vi "Load Views.vi"(8 "error in (no error)":errorcluster, 9 "Views":refnum<class "Actor.lvclass">[](array[class]), 10 "Names":string[](array[string]), 11 "MVVM Abstruct Controller in":refnum<class "MVVM Abstruct Controller.lvclass">) -> (0 "error out":errorcluster, 3 "MVVM Abstruct Controller out":refnum<class "MVVM Abstruct Controller.lvclass">)   [LabVIEW 2020, in "MVVM Abstruct Controller.lvlib" / "MVVM Abstruct Controller.lvclass"]
uses:
  MVVM Abstruct Controller.lvclass
  C:/Program Files (x86)/National Instruments/LabVIEW 2020/vi.lib/ActorFramework/Actor/Actor.lvclass
  <vilib>/ActorFramework/Actor/Actor.lvclass
  MVVM Abstruct Controller.lvclass/MVVM Abstruct Controller.ctl
  C:/Users/yu/Desktop/Pro1/06 Source/Code/Common/ActorMap/ActorMap.lvclass
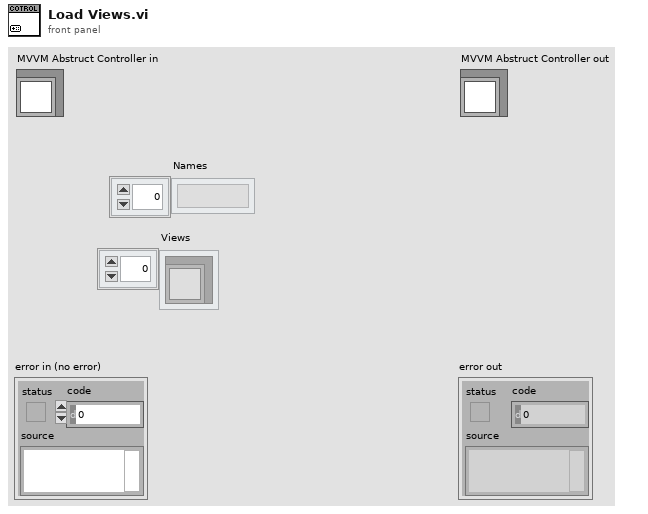
[diagram p1: front panel]
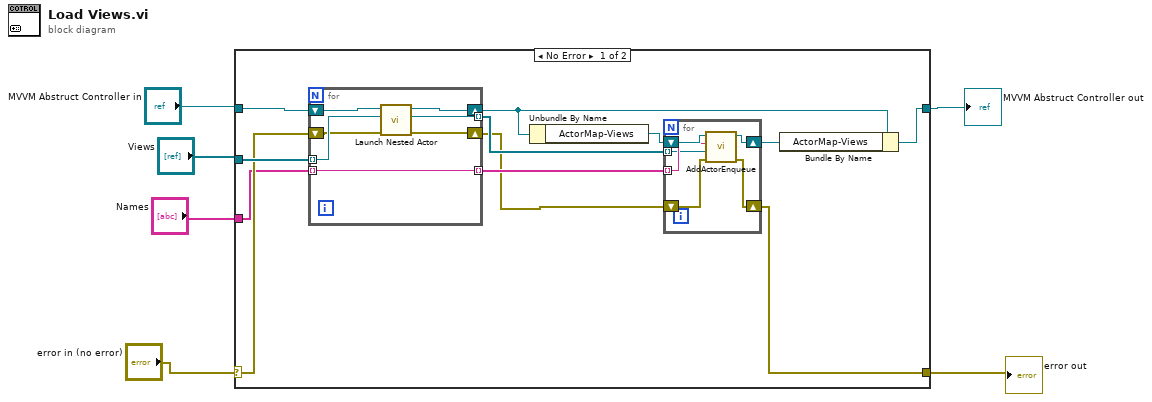
[diagram p0: block diagram]
diagram:
  n1 = case shown="No Error" "error in (no error)" {
    selector: "error in (no error)" -> [w16 w33]
    tunnel: [w8 w33] -> w4
    tunnel: [w7 w32] -> w5
    tunnel: "MVVM Abstruct Controller in" -> [w18 w32]
    tunnel: "Views" -> [w17 _]
    tunnel: "Names" -> [w15 _]
    frame No Error {
      n2 = for {
        shift-right: [w30] -> w10
        shift-left: w18 -> [w31]
        tunnel: w17 -> [w29] mode=indexing
        shift-right: [w27] -> w11
        shift-left: w16 -> [w28]
        tunnel: w15 -> [w26] mode=indexing
        tunnel: [w26] -> w13 mode=indexing
        tunnel: [w25] -> w12 mode=indexing
        n3 = call <vilib>:"Launch Nested Actor.vi"("error in (no error)"=w28, "Nested Actor"=w29, "Caller Actor in"=w31) -> ("error out"=w27:errorcluster, "Nested Actor's Enqueuer"=w25:refnum<class "Message Enqueuer.lvclass">, "Caller Actor out"=w30:refnum<class "MVVM Abstruct Controller.lvclass">)  [unwired: 6 in]
      }
      n4 = Unbundle By Name(w10) -> ("ActorMap-Views"=w14:refnum<class "ActorMap.lvclass">)
      n5 = for {
        tunnel: w13 -> [w23] mode=indexing
        tunnel: w12 -> [w22] mode=indexing
        shift-right: [w21] -> w9
        shift-left: w14 -> [w24]
        shift-right: [w19] -> w8
        shift-left: w11 -> [w20]
        n6 = call "AddActorEnqueue.vi"("error in (no error)"=w20, "Actor's Enqueuer"=w22, "name"=w23, "ActorMap in"=w24) -> ("error out"=w19:errorcluster, "ActorMap out"=w21:refnum<class "ActorMap.lvclass">)  [unwired: 6 in]
      }
      n7 = Bundle By Name(cluster=w10, "ActorMap-Views"=w9) -> (w7:refnum<class "MVVM Abstruct Controller.lvclass">)
    }
    frame Error {
    }
  }
  "error out" <- w4
  "MVVM Abstruct Controller out" <- w5
